vi "SubPanel Guest_Example Message.vi"(0 "Actor Template In":refnum<class "SubPanel Guest.lvclass">, 5 "Response Size":u32, 11 "error in (no error)":errorcluster) -> (4 "Actor Template Out":refnum<class "SubPanel Guest.lvclass">, 6 "Response":string, 15 "error out":errorcluster)   [LabVIEW 2013, in "SubPanel Guest.lvclass"]
uses:
  SubPanel Guest.lvclass
  Actor/src/Connector/FTW-ActorConnector.lvclass
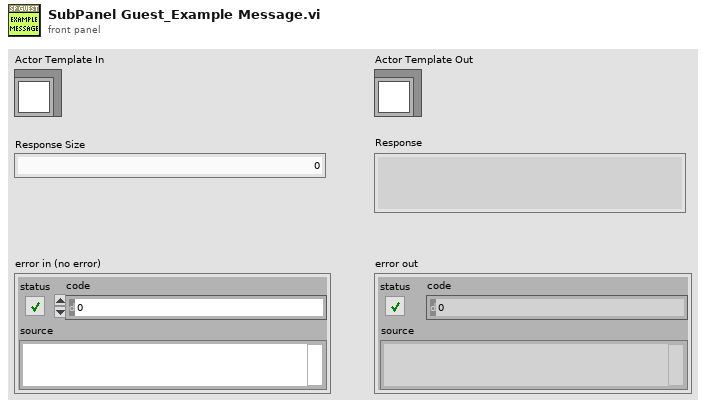
[diagram p1: front panel]
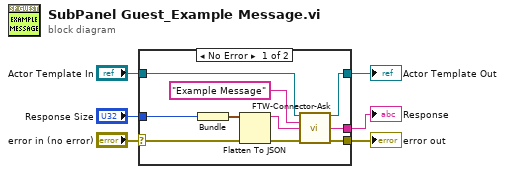
[diagram p0: block diagram]
diagram:
  n1 = case shown="No Error" "error in (no error)" {
    selector: "error in (no error)" -> [w14 w17]
    tunnel: "Actor Template In" -> [w16 w18]
    tunnel: [w15 w18] -> w4
    tunnel: [w13 w17] -> w3
    tunnel: [w10 _] -> w2
    tunnel: "Response Size" -> [w9 _]
    frame No Error {
      n2 = Bundle("Response Size"=w9) -> (w8:cluster{"Response Size":u32})  [unwired: 1 in]
      n3 = Flatten To JSON(anything=w8, error in (no error)=w14) -> (JSON string=w7:string, 11:w11:errorcluster)  [unwired: 1 in]
      n4 = call "FTW-Connector-Ask.vi"("FTW Actor Connector"=w16, "Request Header"="Example Message", "Request Body"=w7, "error in"=w11) -> ("FTW Actor Connector out"=w15:refnum<class "SubPanel Guest.lvclass">, "Response Body"=w10:string, "error out"=w13:errorcluster)  [unwired: 6 in, 3 out]
    }
    frame Error {
    }
  }
  "Actor Template Out" <- w4
  "error out" <- w3
  "Response" <- w2
